vi "Register for Folder Path.vi"(8 "error in (no error)":errorcluster, 11 "File Explorer in":refnum<class "File Explorer.lvclass">) -> (0 "error out":errorcluster, 3 "File Explorer out":refnum<class "File Explorer.lvclass">)   [LabVIEW 2019, in "File Explorer.lvlib" / "File Explorer.lvclass"]
doc: "<RequiredOverrideReason>Use this VI to register for Path to top level folder, or to hardcode the top level folder, whatever you want\nIf you use it to register then be sure to handle the registration in your code</RequiredOverrideReason>"
uses:
  <vilib>/gpm_packages/@cs/file-explorer-extension/Source/File Explorer/File Explorer/File Explorer.lvclass
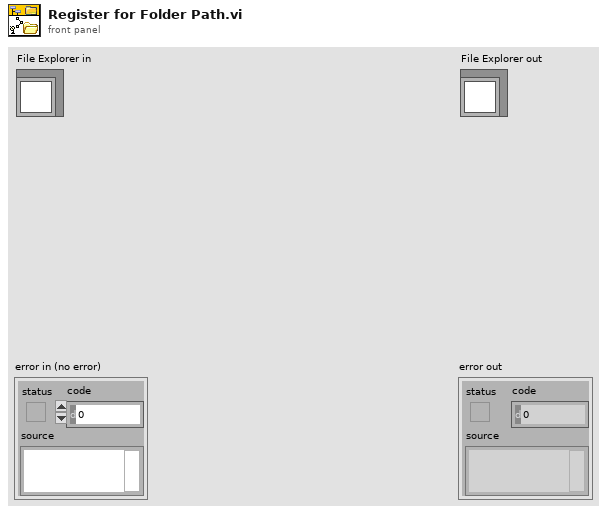
[diagram p1: front panel]
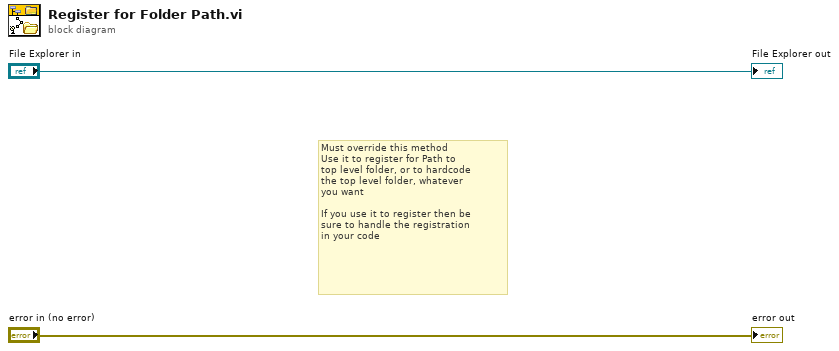
[diagram p0: block diagram]
diagram:
  # "Must override this method\nUse it to register for Path to \ntop level folder, or to hardcode\nthe top level folder, whatever\nyou want\n\nIf you use it to register then be\nsure to handle the registration \nin your code"
  "error out" <- "error in (no error)"
  "File Explorer out" <- "File Explorer in"
